vi "Read From Protected Connection.vi"(8 "error in (no error)":errorcluster, 10 "ProtectedConnectionReader":refnum<class "ProtectedConnectionReader.lvclass">, 11 "IReadPolicy in":refnum<class "ReadStrategy.lvclass">) -> (0 "error out":errorcluster, 2 "Packet":refnum<class "IPacket.lvclass">)   [LabVIEW 2020, in "Network Messenger.lvlib" / "ReadStrategy.lvclass"]
uses:
  <vilib>/gpm_packages/@cs/Network-interface/Source/Network Messenger/ReadStrategy/ReadStrategy.lvclass
  <vilib>/gpm_packages/@cs/Network-interface/Source/ProtectedConnectionReader/ProtectedConnectionReader.lvclass
  <vilib>/gpm_packages/@cs/Network-interface/Source/MessagingInterfaces/IPacket/IPacket.lvclass
  <vilib>/gpm_packages/@cs/Network-interface/Source/ProtectedConnectionReader/ProtectedConnectionReader.lvclass/ProtectedConnectionReader.ctl
  <vilib>/gpm_packages/@cs/Network-interface/Source/Connection Reference/Connection Reference/Connection Reference.lvclass/Connection Reference.ctl
  <vilib>/gpm_packages/@cs/Network-interface/Source/Network Messenger/Types/Message Packet.ctl
  <vilib>/gpm_packages/@cs/Network-interface/Source/Network Messenger/ReadStrategy/Check for Timeout.vi
  <vilib>/gpm_packages/@cs/Network-interface/Source/Network Messenger/ClusterMessagePacket/ClusterMessagePacket.lvclass
  C:/Program Files/National Instruments/LabVIEW 2020/vi.lib/gpm_packages/@cs/Network-interface/Source/MessagingInterfaces/IPacket/IPacket.lvclass
  <vilib>/Utility/error.llb/Error Cluster From Error Code.vi
  <vilib>/gpm_packages/@cs/Network-interface/Source/Connection Reference/IConnection/IConnection.lvclass
  <vilib>/gpm_packages/@cs/Network-interface/Source/Network Messenger/Network Messenger.lvlib
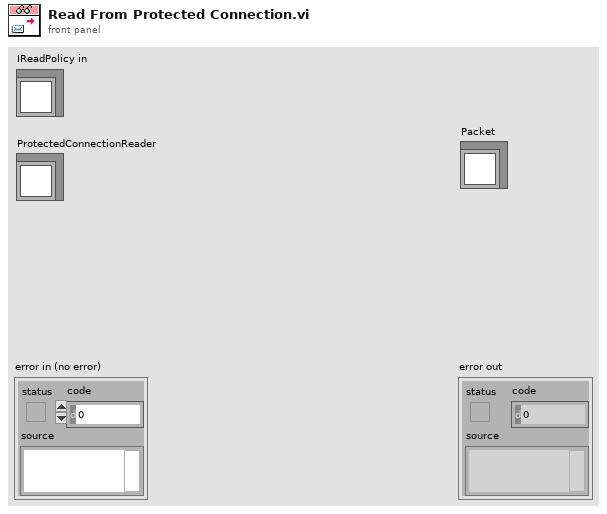
[diagram p1: front panel]
types:
  T1 = typedef "Network Messenger.lvlib/Message Packet.ctl" = cluster{"Msg":string, "Data":variant}
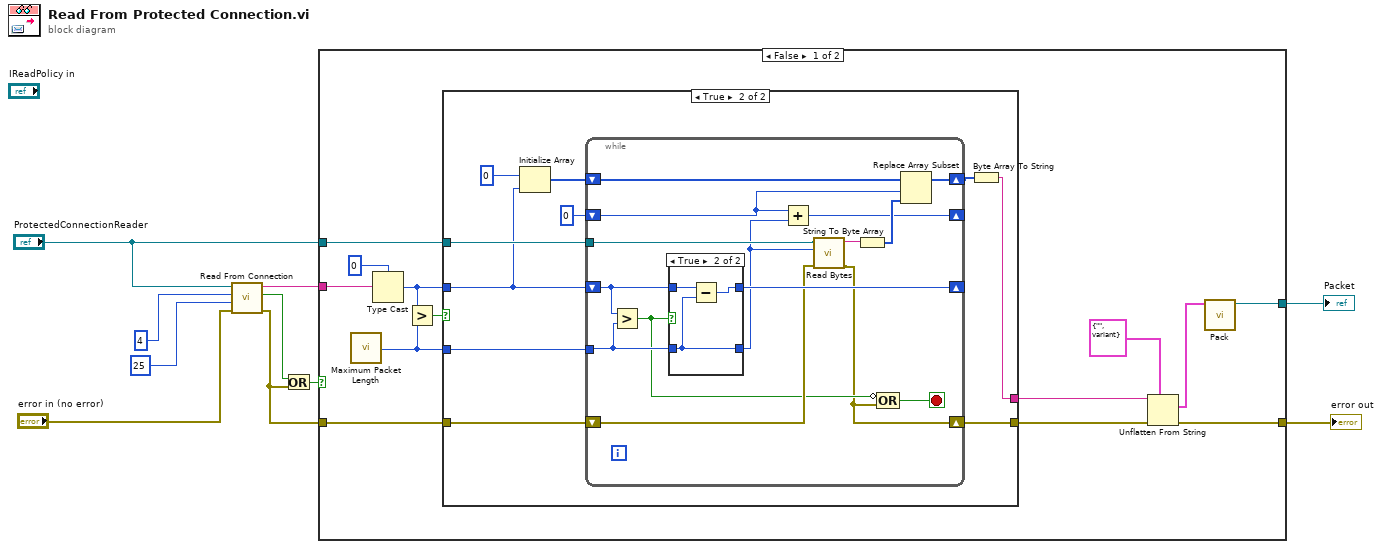
[diagram p0: block diagram]
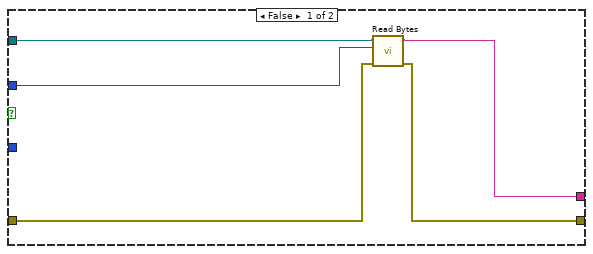
[diagram p2: hidden frame]
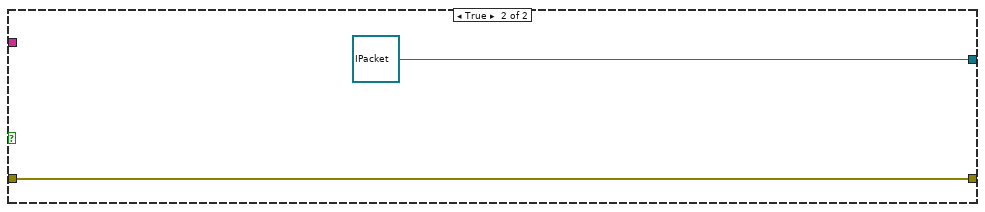
[diagram p4: hidden frame]
diagram:
  n1 = call <vilib>:"Read From Connection.vi"("error in (no error)"="error in (no error)", "Timeout (ms)"=25, "Bytes to Read"=4, "ProtectedConnectionReader in"="ProtectedConnectionReader") -> ("error out"=w7:errorcluster, "TimeOut?"=w6:bool, "Data"=w4:string)  [unwired: 5 in]
  n2 = Or(x=w6, y=w7) -> (x .or. y?=w5:bool)
  n3 = case shown="False" w5 {
    tunnel: w7 -> [w20 w59]
    tunnel: w4 -> [w22 _]
    tunnel: "ProtectedConnectionReader" -> [w23 _]
    tunnel: [w16 w59] -> w2
    tunnel: [w14 refnum<class "IPacket.lvclass"> refnum ("Packet")] -> w1
    frame False {
      n4 = call <vilib>:"Maximum Packet Length.vi"() -> ("Max Packet Length"=w11:i32)
      n5 = Type Cast(type=0, x=w22) -> (*(type *) &x=w12:i32)
      n6 = Greater?(x=w12, y=w11) -> (0:w13:bool)
      n7 = case shown="True" w13 {
        tunnel: w23 -> [w28 w38]
        tunnel: w12 -> [w24 w33]
        tunnel: w20 -> [w26 w37]
        tunnel: [w25 w35] -> w19
        tunnel: [w27 w30] -> w18
        tunnel: w11 -> [_ w36]
        frame False {
          n8 = call <vilib>:"Read Bytes.vi"("error in (no error)"=w26, "Bytes to Read"=w24, "ProtectedConnectionReader"=w28) -> ("error out"=w25:errorcluster, "Message"=w27:string)  [unwired: 7 in]
        }
        frame True {
          n9 = Initialize Array(u8 0 ("element"), w33) -> (w32:u8[])
          n10 = while {
            tunnel: w38 -> [w44]
            shift-right: [w39] -> w35
            shift-left: w37 -> [w45]
            tunnel: w36 -> [w51]
            shift-right: [w53] -> _
            shift-left: w33 -> [w52]
            shift-right: [w49] -> w31
            shift-left: w32 -> [w50]
            shift-right: [w46] -> _
            shift-left: 0 -> [w47]
            stop <- w40 stop-if-true
            n11 = Greater?(x=w52, y=w51) -> (0:w41:bool)
            n12 = case shown="True" w41 {
              tunnel: [_ w57] -> w53
              tunnel: w52 -> [w54 w56]
              tunnel: w51 -> [_ w55]
              tunnel: [w54 w55] -> w42
              frame False {
              }
              frame True {
                n13 = Subtract(x=w56, y=w55) -> (x-y=w57:i32)
              }
            }
            n14 = Add(x=w47, y=w42) -> (x+y=w46:i32)
            n15 = call <vilib>:"Read Bytes.vi"("error in (no error)"=w45, "Bytes to Read"=w42, "ProtectedConnectionReader"=w44) -> ("error out"=w39:errorcluster, "Message"=w43:string)  [unwired: 7 in]
            n16 = String To Byte Array(string=w43) -> (unsigned byte array=w48:u8[])
            n17 = Compound Arithmetic op=OR(invert w41, w39) -> (w40:bool)
            n18 = Replace Array Subset(array=w50, new element=w48, index=w47) -> (w49:u8[])
          }
          n19 = Byte Array To String(unsigned byte array=w31) -> (string=w30:string)
        }
      }
      n20 = Unflatten From String(type=T1 {"Msg"="", "Data"=variant}, binary string=w18, error in (no error)=w19) -> (value=w15:T1, error out=w16:errorcluster)  [unwired: 2 in, 1 out]
      n21 = call <vilib>:"Pack.vi"("Packet"=w15) -> ("ClusterMessagePacket out"=w14:refnum<class "ClusterMessagePacket.lvclass">)  [unwired: 10 in]
    }
    frame True {
    }
  }
  "error out" <- w2
  "Packet" <- w1
